vi "FrontPanel.vi"() -> ()   [LabVIEW 2009]
panel:
  in  "Tab Control":enum32{"Page 1", "Page 2", "Page 3", "Page 4"}(tab)
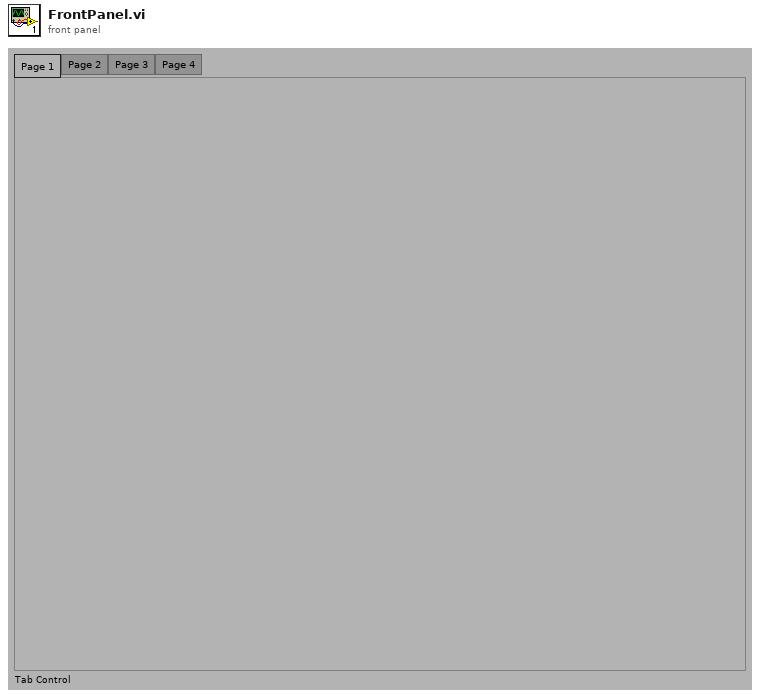
[diagram p1: front panel]
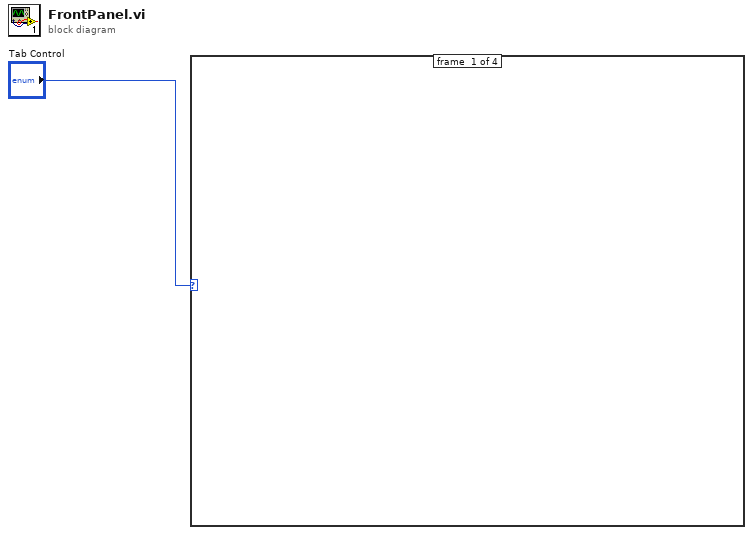
[diagram p0: block diagram]
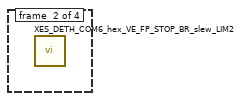
[diagram p2: hidden frame]
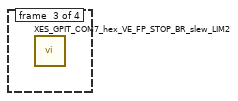
[diagram p3: hidden frame]
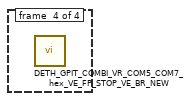
[diagram p4: hidden frame]
diagram:
  n1 = case shown="\"Page 3\"" "Tab Control" {
    frame #0 {
    }
    frame #1 {
      n2 = call "XES_DETH_COM6_hex_VE_FP_STOP_BR_slew_LIM2.vi"() -> ()  [unwired: 1 in]
    }
    frame #2 {
      n3 = call "XES_GPIT_COM7_hex_VE_FP_STOP_BR_slew_LIM2.vi"() -> ()  [unwired: 1 in]
    }
    frame #3 {
      n4 = call "DETH_GPIT_COMBI_VR_COM5_COM7_hex_VE_FP_STOP_VE_BR_NEW.vi"() -> ()  [unwired: 1 in]
    }
  }
